vi "Update Bind Methods.vi"(8 "error in (no error)":errorcluster, 10 "RPC Method Parameters":T1, 11 "Server class in":refnum<vi>) -> (0 "error out":errorcluster, 3 "Server class out":refnum<vi>)   [LabVIEW 2019, in "gRPC Template Creation Utility.lvlib"]
uses:
  gRPC Template Creation Utility.lvlib
  TypeDefs/RPC Method Parameters.ctl
  <vilib>/Utility/error.llb/Trim Whitespace One-Sided.vi
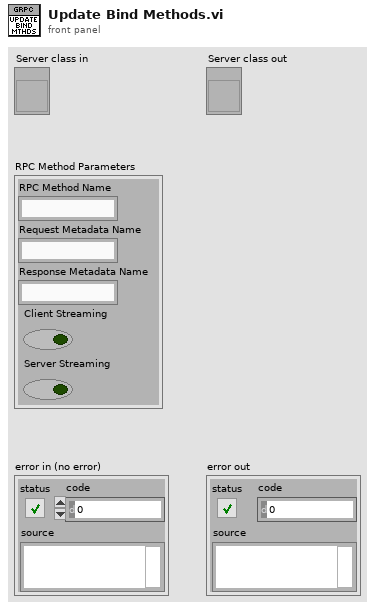
[diagram p1: front panel]
types:
  T1 = typedef "gRPC Template Creation Utility.lvlib/RPC Method Parameters.ctl" = cluster{"RPC Method Name":string, "Request Metadata Name":string, "Response Metadata Name":string, "Client Streaming":bool, "Server Streaming":bool}
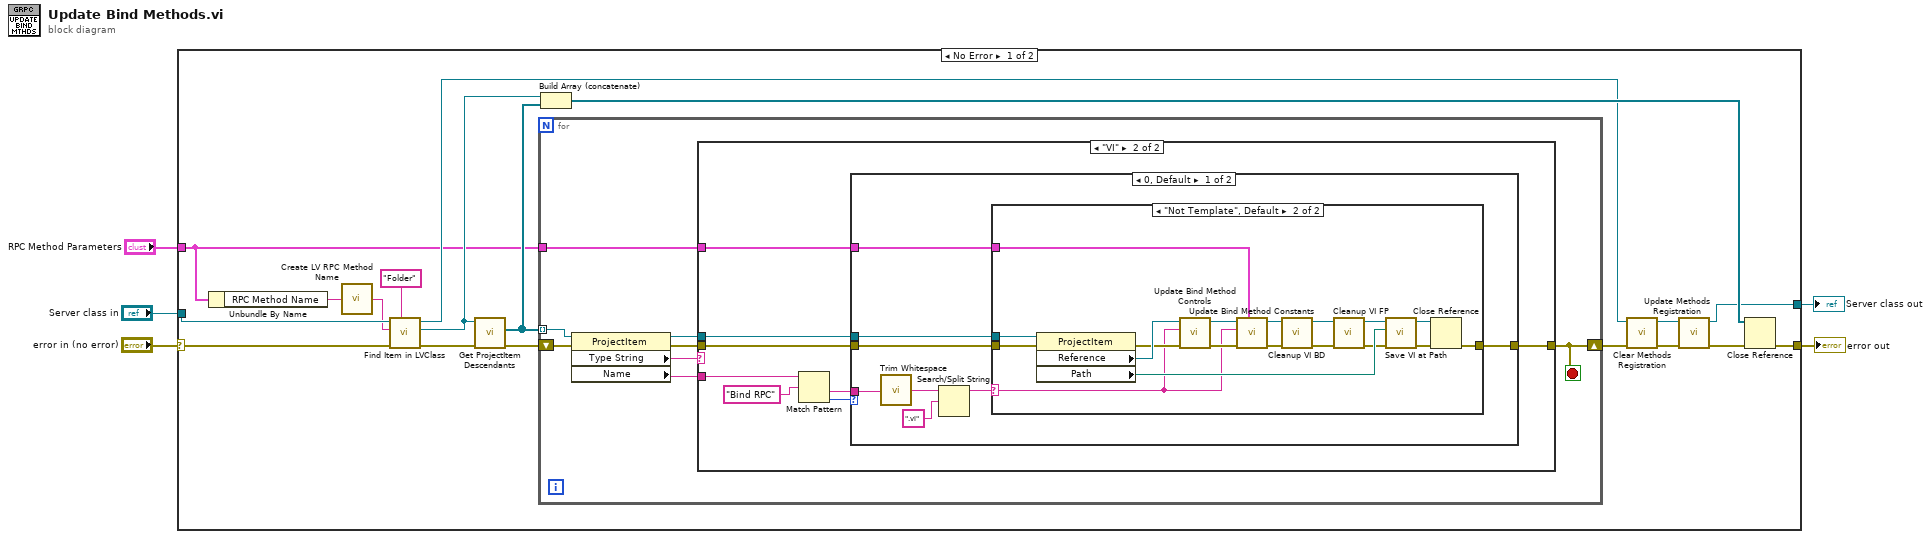
[diagram p0: block diagram]
diagram:
  n1 = case shown="No Error" "error in (no error)" {
    selector: "error in (no error)" -> [w16 w70]
    tunnel: [w10 w70] -> w5
    tunnel: "Server class in" -> [w18 w69]
    tunnel: [w9 w69] -> w2
    tunnel: "RPC Method Parameters" -> [w8 _]
    frame No Error {
      n2 = Unbundle By Name(w8) -> ("RPC Method Name"=w7:string)
      n3 = call "Create LV RPC Method Name.vi"("Proto Parser RPC Method Name in"=w7) -> ("LV RPC Method Name out"=w6:string)
      n4 = call "Find Item in LVClass.vi"("Item Type"="Folder", "error in (no error)"=w16, "Item Name"=w6, "Class Item in"=w18) -> ("error out"=w19:errorcluster, "Project Item (Class Item)"=w20:refnum<vi>, "Class Item out"=w12:refnum<vi>)  [unwired: 4 in, 1 out]
      n5 = call "Get ProjectItem Descendants.vi"("error in (no error)"=w19, "ProjectItem in"=w20) -> ("error out"=w23:errorcluster, "All Descendents"=w21:refnum<vi>[])  [unwired: 7 in, 1 out]
      n6 = for {
        tunnel: w21 -> [w31] mode=indexing
        shift-right: [w25] -> w13
        shift-left: w23 -> [w28]
        tunnel: w8 -> [w24]
        stop <- w25 stop-if-true
        n7 = property class="ProjectItem"(reference=w31, error in=w28) -> (reference out=w29:refnum<vi>, error out=w27:errorcluster, "Type String"=w30:string, "Name"=w26:string)
        n8 = case shown="\"VI\"" w30 {
          tunnel: w29 -> [_ w38]
          tunnel: w27 -> [w32 w36]
          tunnel: w26 -> [_ w34]
          tunnel: [w32 w37] -> w25
          tunnel: w24 -> [_ w33]
          frame "None", Default {
          }
          frame "VI" {
            n9 = Match Pattern(string=w34, regular expression="Bind RPC") -> (after substring=w35:string, offset past match=w39:i32)  [unwired: 1 in, 2 out]
            n10 = case shown="0, Default" w39 {
              tunnel: w38 -> [w48 _]
              tunnel: [w46 w68] -> w37
              tunnel: w36 -> [w47 w68]
              tunnel: w35 -> [w45 _]
              tunnel: w33 -> [w41 _]
              frame 0, Default {
                n11 = call <vilib>:"Trim Whitespace.vi"("string"=w45) -> ("trimmed string"=w44:string)  [unwired: 1 in]
                n12 = Search/Split String(string=w44, search string/char (-)=".vi" ("regular expression")) -> (substring before match=w42:string)  [unwired: 1 in, 2 out]
                n13 = case shown="\"Not Template\", Default" w42 {
                  selector: w42 -> [_ w57]
                  tunnel: w48 -> [_ w67]
                  tunnel: w47 -> [w49 w66]
                  tunnel: [w49 w61] -> w46
                  tunnel: w41 -> [_ w56]
                  frame "package_service_method" {
                  }
                  frame "Not Template", Default {
                    n14 = property class="ProjectItem"(reference=w67, error in=w66) -> (error out=w64:errorcluster, "Reference"=w65:refnum<vi>, "Path"=w58:path)  [unwired: 1 out]
                    n15 = call "Update Bind Method Controls.vi"("error in (no error)"=w64, "Method Name"=w57, "VI in"=w65) -> ("error out"=w63:errorcluster, "VI out"=w62:refnum<vi>)  [unwired: 7 in]
                    n16 = call "Update Bind Method Constants.vi"("RPC Method Parameters"=w56, "error in (no error)"=w63, "RPC Method Name"=w57, "VI in"=w62) -> ("error out"=w51:errorcluster, "VI out"=w53:refnum<vi>)  [unwired: 6 in]
                    n17 = call "Cleanup VI BD.vi"("error in (no error)"=w51, "VI in"=w53) -> ("error out"=w55:errorcluster, "VI out"=w54:refnum<vi>)  [unwired: 8 in]
                    n18 = call "Cleanup VI FP.vi"("error in"=w55, "vi in"=w54) -> ("error out"=w50:errorcluster, "vi out"=w52:refnum<vi>)  [unwired: 8 in]
                    n19 = call "Save VI at Path.vi"("error in (no error)"=w50, "Path"=w58, "VI in"=w52) -> ("error out"=w60:errorcluster, "VI out"=w59:refnum<vi>)  [unwired: 6 in, 1 out]
                    n20 = Close Reference(reference=w59, error in (no error)=w60) -> (error out=w61:errorcluster)
                  }
                }
              }
              frame -1 {
              }
            }
          }
        }
      }
      n21 = Build Array (concatenate)(w20, w21) -> (w22:refnum<vi>[])
      n22 = call "Clear Methods Registration.vi"("error in (no error)"=w13, "Server class in"=w12) -> ("error out"=w15:errorcluster, "Server class out"=w14:refnum<vi>)  [unwired: 8 in]
      n23 = call "Update Methods Registration.vi"("error in (no error)"=w15, "Server class in"=w14) -> ("error out"=w11:errorcluster, "Server class out"=w9:refnum<vi>)  [unwired: 8 in]
      n24 = Close Reference(reference=w22, error in (no error)=w11) -> (error out=w10:errorcluster)
    }
    frame Error {
    }
  }
  "error out" <- w5
  "Server class out" <- w2
